vi "Odd_or_Even.vi"() -> ()   [LabVIEW 2020]
panel:
  out "Odd":bool
  out "Even":bool
  in  "Number":dbl
  # "Find whether the given number is odd or even"
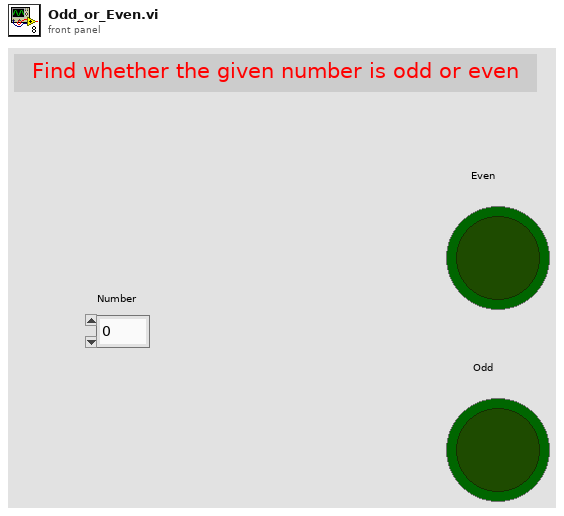
[diagram p1: front panel]
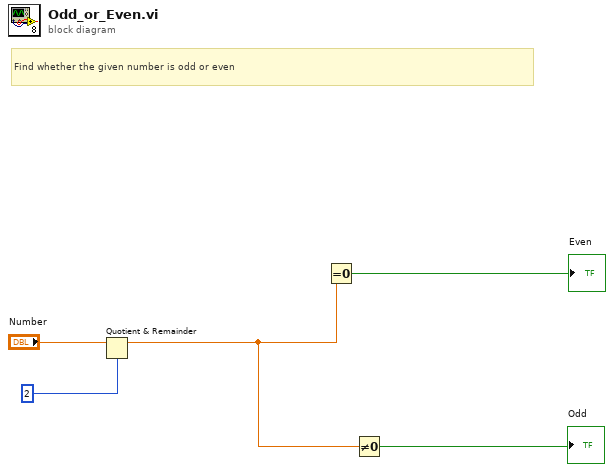
[diagram p0: block diagram]
diagram:
  # "Find whether the given number is odd or even"
  n1 = Quotient & Remainder(x="Number", y=2) -> (x-y*floor(x/y)=w1:dbl)  [unwired: 1 out]
  n2 = Equal To 0?(x=w1) -> (x = 0?=→"Even":bool)
  n3 = Not Equal To 0?(x=w1) -> (x != 0?=→"Odd":bool)
